vi "Get Full Name.vi"(11 "CIFPluginLoader in":refnum<class "CIFPluginLoader.lvclass">) -> (3 "Full Name":string)   [LabVIEW 2021, in "CIFPluginLoader.lvclass"]
uses:
  CIFPluginLoader.lvclass
  CIFPluginLoader.lvclass/CIFPluginLoader.ctl
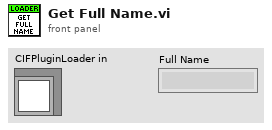
[diagram p1: front panel]
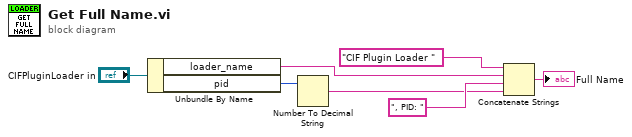
[diagram p0: block diagram]
diagram:
  n1 = Unbundle By Name("CIFPluginLoader in") -> ("loader_name"=w4:string, "pid"=w5:u32)
  n2 = Number To Decimal String(number=w5) -> (decimal integer string=w6:string)  [unwired: 1 in]
  n3 = Concatenate Strings("CIF Plugin Loader " ("message"), w4, ", PID: " ("message"), w6) -> (→"Full Name":string)
